vi "toOCU.vi"(8 "error in (no error)":errorcluster, 10 "NotifierReff":T1, 11 "NetworkStreamWriter in":refnum<class "NetworkStreamWriter.lvclass">) -> (0 "error out":errorcluster, 3 "NetworkStreamWriter out":refnum<class "NetworkStreamWriter.lvclass">)   [LabVIEW 2013]
doc: "writes all notifiers to OCU when they're updated\n\nImportaint: when new notifiers are created, this VI must be updated. For doubles, booleans, and double arrays, simply add them to the appropriate unbundle category. For anything else, add them to the \"other\" category and copy the code from the others.\n\nKaitlin Gallagher\n3/4/14"
uses:
  RIO-OCU_Comm/NetworkStreams/Writer/NetworkStreamWriter.lvclass
  Data/TypeDefs/Notifiers.ctl
  Data/TypeDefs/UTM Location.ctl
  Data/TypeDefs/Sail Set Suggestions.ctl
  Data/TypeDefs/Rudder Set Suggestions.ctl
  Data/TypeDefs/OverrideInformation.ctl
  Data/TypeDefs/OverrideMode.ctl
  Data/TypeDefs/MotorSetup.ctl
  Data/TypeDefs/DynamixelSetupInfo.ctl
  Data/TypeDefs/AirmarStatus.ctl
  Data/TypeDefs/HardwareOnline.ctl
  <vilib>/Utility/VariantDataType/VariantType.lvlib
panel:
  out "error in (no error) 3":errorcluster
  in  "error in (no error) 2":errorcluster
  out "latest notification":dbl
  out "Numeric":i32
  out "Array":string[](array[string])
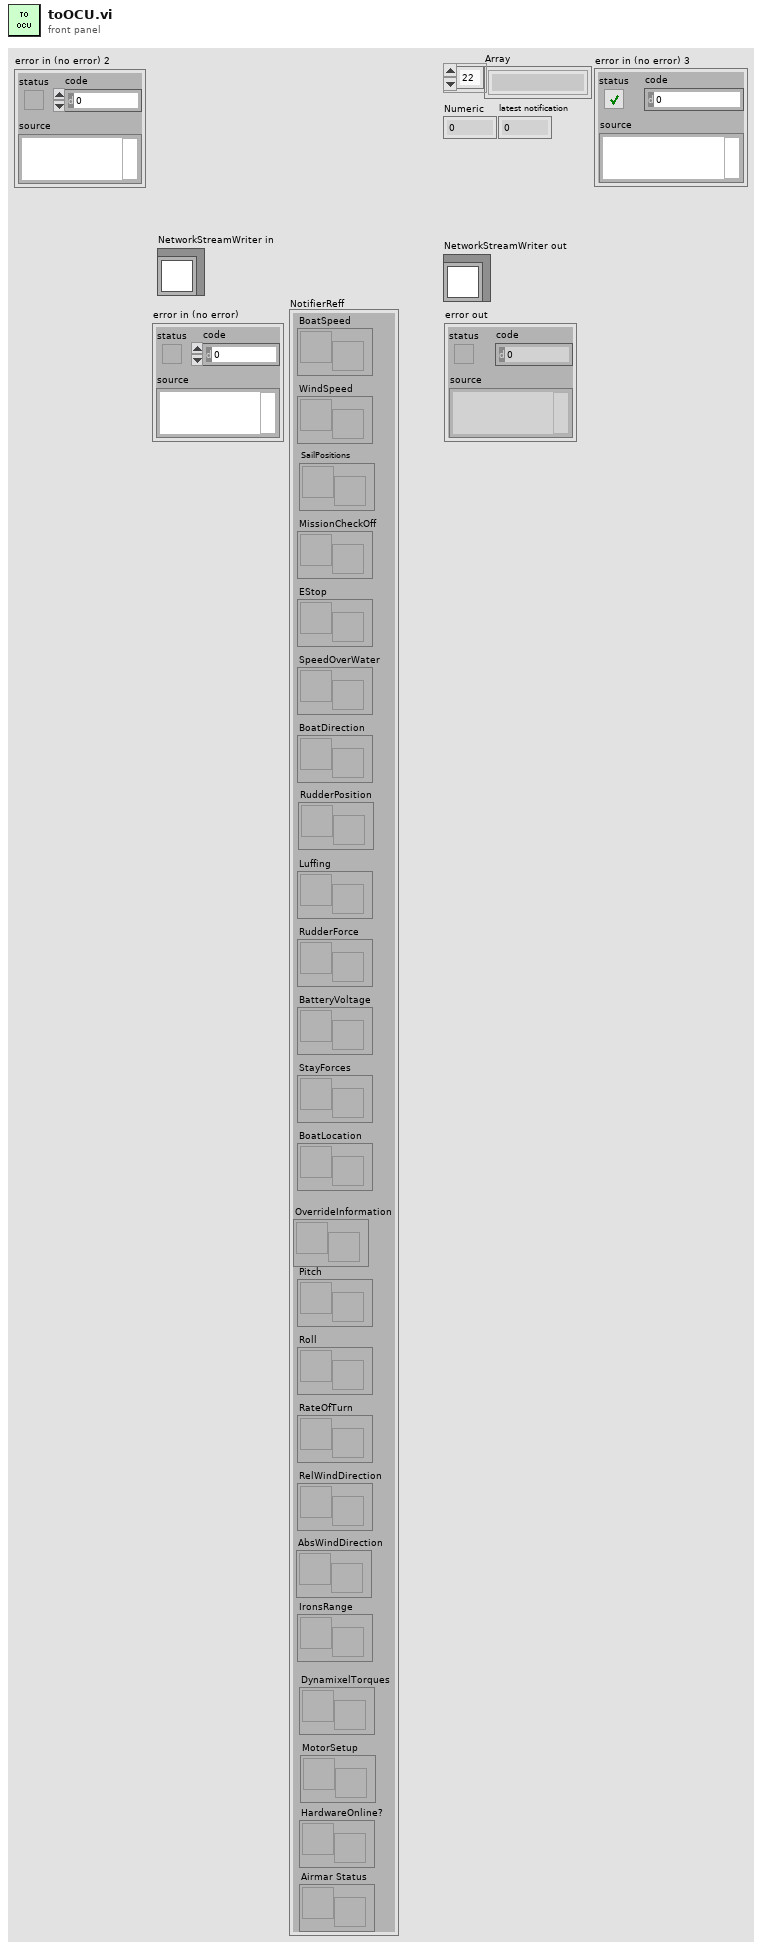
[diagram p1: front panel]
types:
  T1 = typedef "Notifiers.ctl" = cluster{"BoatSpeed":refnum<notifier>, "WindSpeed":refnum<notifier>, "MissionCheckOff":refnum<notifier>, "EStop":refnum<notifier>, "SpeedOverWater":refnum<notifier>, "BoatDirection":refnum<notifier>, "Luffing":refnum<notifier>, "RudderForce":refnum<notifier>, "BatteryVoltage":refnum<notifier>, "StayForces":refnum<notifier>, "BoatLocation":refnum<notifier>, "Pitch":refnum<notifier>, "Roll":refnum<notifier>, "RateOfTurn":refnum<notifier>, "RelWindDirection":refnum<notifier>, "SailPositions":refnum<notifier>, "RudderPosition":refnum<notifier>, "IronsRange":refnum<notifier>, "AbsWindDirection":refnum<notifier>, "OverrideInformation":refnum<notifier>, "DynamixelTorques":refnum<notifier>, "MotorSetup":refnum<notifier>, "Airmar Status":refnum<notifier>, "HardwareOnline?":refnum<notifier>}
  T2 = typedef "HardwareOnline.ctl" = cluster{"AirmarOnline":bool, "WindvaneOnline":bool, "HemisphereOnline":bool, "StayForceOnline":bool, "BatteryVoltageOnline":bool, "AccelerometerOnline":bool, "MainDynamixel Online":bool, "JibDynamixel Online":bool, "RudderDynamixel Online":bool}
  T3 = typedef "MotorSetup.ctl" = cluster{"Main Dynamixel Set Data":T4, "Rudder Dynamixel Set Data":T4, "Jib Dynamixel Set Data":T4}
  T4 = typedef "DynamixelSetupInfo.ctl" = cluster{"Lower Winch Bound":dbl, "Upper Winch Bound":dbl, "Reverse Winch Direction?":bool, "Dynamixel Cycle Number":i32}
  T5 = typedef "OverrideInformation.ctl" = cluster{"OverrideMode":T6, "SailSetting":T7, "Rudder Setpoint":T8}
  T6 = typedef "OverrideMode.ctl" = enum16{"None", "Rudder", "Sails", "Both"}
  T7 = typedef "Sail Set Suggestions.ctl" = cluster{"MainSailSuggestion":dbl, "JibSailSuggestion":dbl}
  T8 = typedef "Rudder Set Suggestions.ctl" = dbl
  T9 = typedef "UTM Location.ctl" = cluster{"UTM Zone":dbl, "Hemisphere":enum16{"North", "South"}, "East":dbl, "North":dbl}
  T10 = typedef "VariantType.lvlib/Type.ctl" = enum8{"Invalid Type", "Void", "I8", "I16", "I32", "I64", "U8", "U16", "U32", "U64", "Single Float", "Double Float", "Extended Float", "Single Complex", "Double Complex", "Extended Complex", "Enum U8", "Enum U16", "Enum U32", "Enum U64", "Single Float With Unit", "Double Float With Unit", "Extended Float With Unit", "Single Complex with Unit", "Double Complex with Unit", "Extended Complex with Unit", "Boolean", "String", "Path", "Picture", "Tag", "Array", "Cluster", "Variant", "LV Variant", "Waveform", "Timestamp", "Digital Waveform", "Digital Data", "ExpressData", "Refnum", "External Data", "VI", "Poly VI", "LabVIEW Class Instance", "Fixed Point"}
  T11 = cluster{"AirmarOnline":bool, "WindvaneOnline":bool, "HemisphereOnline":bool, "RudderForceOnline":bool, "StayForceOnline":bool, "BatteryVoltageOnline":bool, "AccelerometerOnline":bool, "MainDynamixel Online":bool, "JibDynamixel Online":bool, "RudderDynamixel Online":bool}
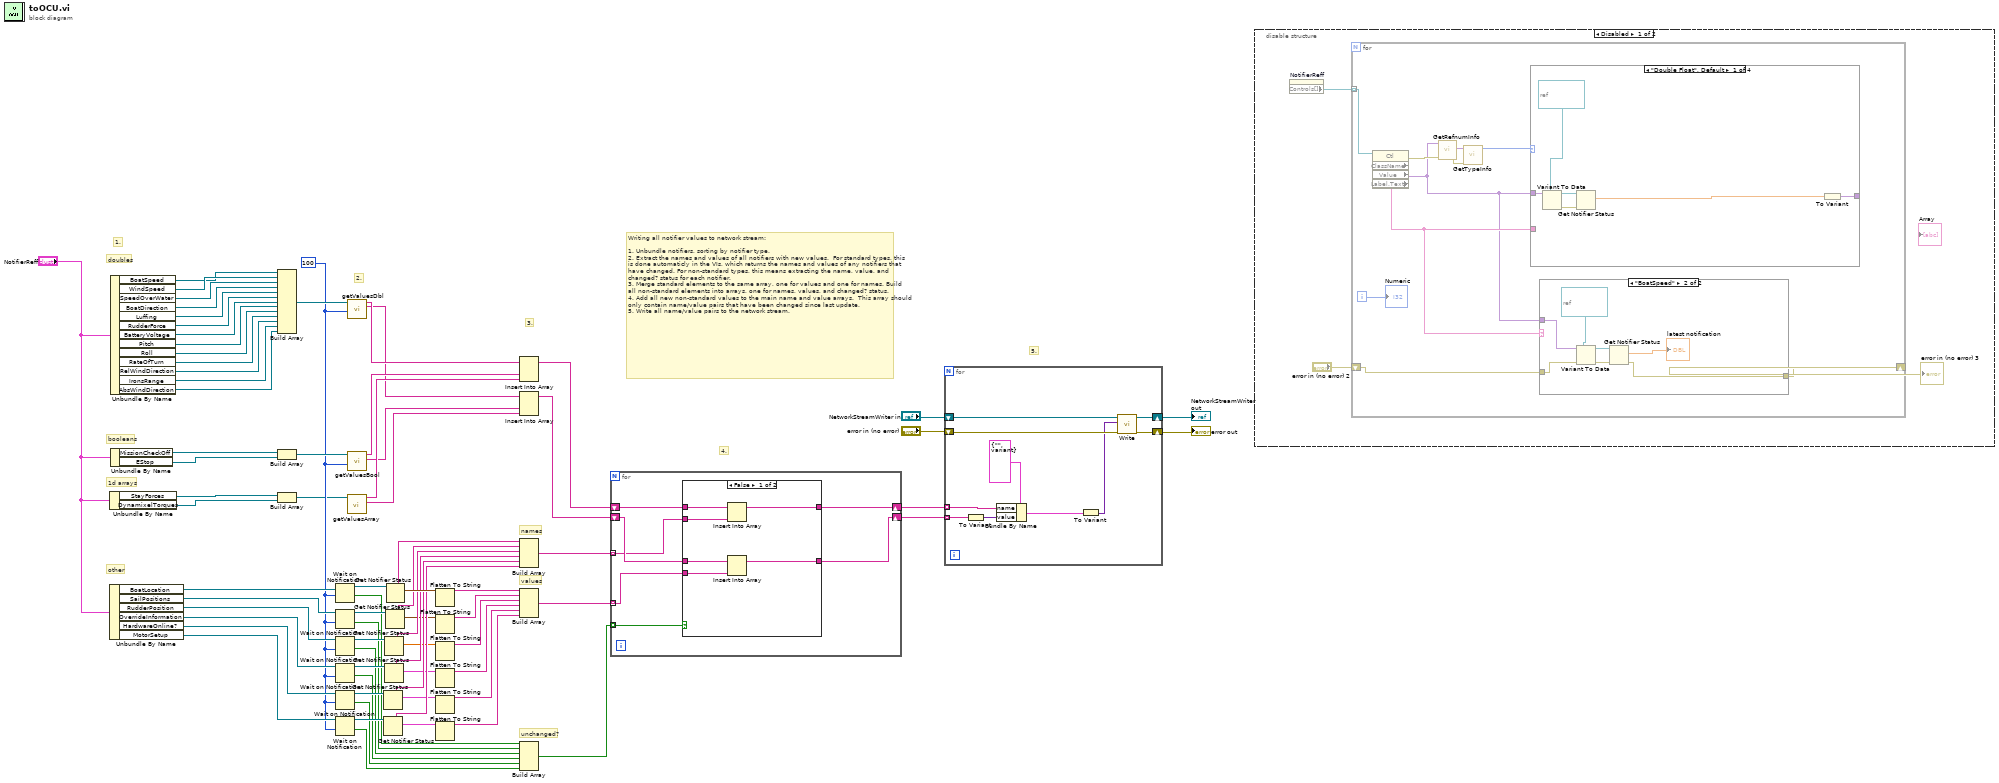
[diagram p0: block diagram]
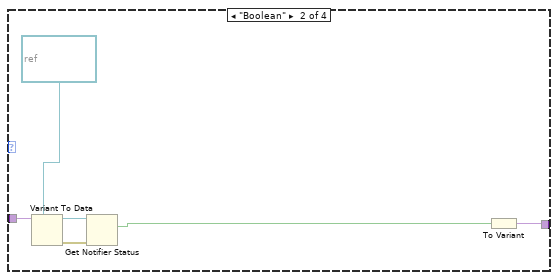
[diagram p3: hidden frame]
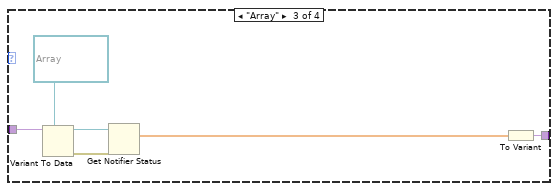
[diagram p4: hidden frame]
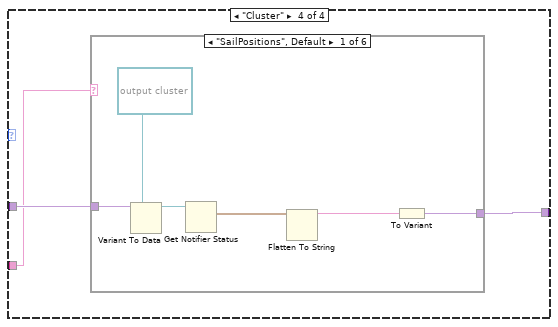
[diagram p5: hidden frame]
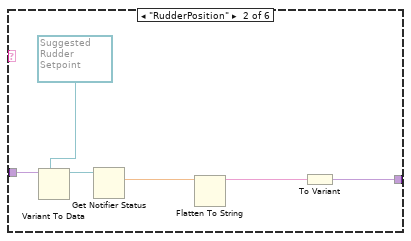
[diagram p6: hidden frame]
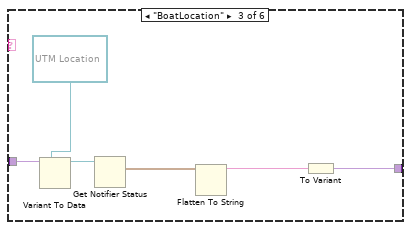
[diagram p7: hidden frame]
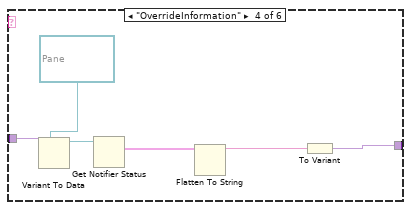
[diagram p8: hidden frame]
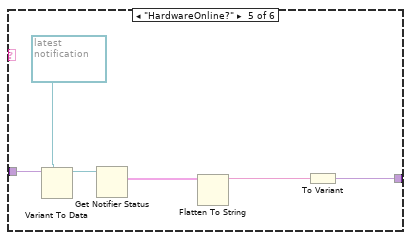
[diagram p9: hidden frame]
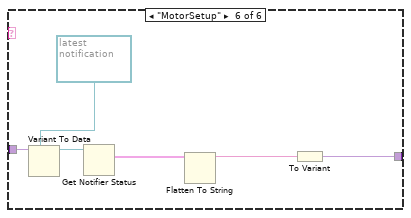
[diagram p10: hidden frame]
diagram:
  w39 = 100 ("timeout in ms (-1)")
  # "Writing all notifier values to network stream:\n\n1. Unbundle notifiers, sorting by notifier type.\n2. Extract the names and values of all notifiers with new values.  For standard types, this is done automaticly in the VIs, which returns the names and values of any notifiers that have changed. For non-standard types, this means extracting the name, value, and changed? status for each notifier. \n3. Merge standard elements to the same array, one for values and one for names. Build all non-standard elements into arrays, one for names, values, and changed? status.\n4. Add all new non-standard values to the main name and value arrays.  This array should only contain name/value pairs that have been changed since last update.\n5. Write all name/value pairs to the network stream."
  # "5."
  # "4."
  # "3."
  # "2."
  # "1."
  # "unchanged?"
  # "values"
  # "names"
  # "other"
  # "1d arrays"
  # "booleans"
  # "doubles"
  n1 = Unbundle By Name("NotifierReff") -> ("StayForces"=w59:refnum<notifier>, "DynamixelTorques"=w62:refnum<notifier>)
  n2 = Unbundle By Name("NotifierReff") -> ("BoatLocation"=w58:refnum<notifier>, "SailPositions"=w57:refnum<notifier>, "RudderPosition"=w56:refnum<notifier>, "OverrideInformation"=w54:refnum<notifier>, "HardwareOnline?"=w55:refnum<notifier>, "MotorSetup"=w53:refnum<notifier>)
  n3 = Unbundle By Name("NotifierReff") -> ("BoatSpeed"=w42:refnum<notifier>, "WindSpeed"=w75:refnum<notifier>, "SpeedOverWater"=w74:refnum<notifier>, "BoatDirection"=w73:refnum<notifier>, "Luffing"=w72:refnum<notifier>, "RudderForce"=w71:refnum<notifier>, "BatteryVoltage"=w70:refnum<notifier>, "Pitch"=w69:refnum<notifier>, "Roll"=w68:refnum<notifier>, "RateOfTurn"=w67:refnum<notifier>, "RelWindDirection"=w66:refnum<notifier>, "IronsRange"=w65:refnum<notifier>, "AbsWindDirection"=w64:refnum<notifier>)
  n4 = Unbundle By Name("NotifierReff") -> ("MissionCheckOff"=w60:refnum<notifier>, "EStop"=w63:refnum<notifier>)
  n5 = Build Array(w42, w75, w74, w73, w72, w71, w70, w69, w68, w67, w66, w65, w64) -> (w41:refnum<notifier>[])
  n6 = Build Array(w60, w63) -> (w40:refnum<notifier>[])
  n7 = Build Array(w59, w62) -> (w38:refnum<notifier>[])
  n8 = Wait on Notification(notifier=w58, timeout in ms (-1)=w39) -> (notifier out=w37:refnum<notifier>, timed out?=w14:bool)  [unwired: 2 in, 2 out]
  n9 = Wait on Notification(notifier=w57, timeout in ms (-1)=w39) -> (notifier out=w34:refnum<notifier>, timed out?=w15:bool)  [unwired: 2 in, 2 out]
  n10 = Wait on Notification(notifier=w56, timeout in ms (-1)=w39) -> (notifier out=w32:refnum<notifier>, timed out?=w16:bool)  [unwired: 2 in, 2 out]
  n11 = Wait on Notification(notifier=w54, timeout in ms (-1)=w39) -> (notifier out=w30:refnum<notifier>, timed out?=w17:bool)  [unwired: 2 in, 2 out]
  n12 = Wait on Notification(notifier=w55, timeout in ms (-1)=w39) -> (notifier out=w28:refnum<notifier>, timed out?=w18:bool)  [unwired: 2 in, 2 out]
  n13 = Wait on Notification(notifier=w53, timeout in ms (-1)=w39) -> (notifier out=w26:refnum<notifier>, timed out?=w19:bool)  [unwired: 2 in, 2 out]
  n14 = call "getValuesArray.vi"("appended array"=w38) -> ("notifier values"=w8:string[], "notifier names"=w11:string[])  [unwired: 8 in, 1 out]
  n15 = call "getValuesDbl.vi"("timeout in ms (-1)"=w39, "notifiers in"=w41) -> ("notifier values"=w10:string[], "notifier names"=w13:string[])  [unwired: 7 in, 1 out]
  n16 = call "getValuesBool.vi"("timeout in ms (-1)"=w39, "notifiers in"=w40) -> ("notifier values"=w9:string[], "notifier names"=w12:string[])  [unwired: 7 in, 1 out]
  n17 = Get Notifier Status(notifier=w28) -> (notifier name=w27:string, current notification=w21:T2)  [unwired: 1 in, 3 out]
  n18 = Get Notifier Status(notifier=w26) -> (notifier name=w25:string, current notification=w20:T3)  [unwired: 1 in, 3 out]
  n19 = Get Notifier Status(notifier=w30) -> (notifier name=w29:string, current notification=w22:T5)  [unwired: 1 in, 3 out]
  n20 = Get Notifier Status(notifier=w32) -> (notifier name=w31:string, current notification=w23:T8)  [unwired: 1 in, 3 out]
  n21 = Get Notifier Status(notifier=w34) -> (notifier name=w33:string, current notification=w24:T7)  [unwired: 1 in, 3 out]
  n22 = Get Notifier Status(notifier=w37) -> (notifier name=w35:string, current notification=w36:T9)  [unwired: 1 in, 3 out]
  n23 = Flatten To String(anything=w36) -> (data string=w52:string)  [unwired: 3 in, 2 out]
  n24 = Flatten To String(anything=w24) -> (data string=w51:string)  [unwired: 3 in, 2 out]
  n25 = Flatten To String(anything=w23) -> (data string=w50:string)  [unwired: 3 in, 2 out]
  n26 = Flatten To String(anything=w22) -> (data string=w49:string)  [unwired: 3 in, 2 out]
  n27 = Flatten To String(anything=w21) -> (data string=w48:string)  [unwired: 3 in, 2 out]
  n28 = Flatten To String(anything=w20) -> (data string=w47:string)  [unwired: 3 in, 2 out]
  n29 = Insert Into Array(array=w13, new element #1=w12, new element #2=w11) -> (w7:string[])  [unwired: 1 in]
  n30 = Insert Into Array(array=w10, new element #1=w9, new element #2=w8) -> (w6:string[])  [unwired: 1 in]
  n31 = Build Array(w35, w33, w31, w29, w27, w25) -> (w4:string[])
  n32 = Build Array(w52, w51, w50, w49, w48, w47) -> (w3:string[])
  n33 = Build Array(w14, w15, w16, w17, w18, w19) -> (w5:bool[])
  n34 = for {
    tunnel: w5 -> [w82] mode=indexing
    shift-right: [w81] -> w2
    shift-left: w7 -> [w76]
    shift-right: [w79] -> w1
    shift-left: w6 -> [w80]
    tunnel: w4 -> [w78] mode=indexing
    tunnel: w3 -> [w77] mode=indexing
    n35 = case shown="False" w82 {
      tunnel: [w88 w89] -> w81
      tunnel: w80 -> [w87 w90]
      tunnel: [w86 w90] -> w79
      tunnel: w78 -> [w85 _]
      tunnel: w77 -> [w84 _]
      tunnel: w76 -> [w83 w89]
      frame False {
        n36 = Insert Into Array(array=w83, new element=w85) -> (w88:string[])  [unwired: 1 in]
        n37 = Insert Into Array(array=w87, new element=w84) -> (w86:string[])  [unwired: 1 in]
      }
      frame True {
      }
    }
  }
  n38 = for {
    shift-right: [w97] -> w43
    shift-left: "error in (no error)" -> [w100]
    shift-right: [w98] -> w44
    shift-left: "NetworkStreamWriter in" -> [w99]
    tunnel: w2 -> [w94] mode=indexing
    tunnel: w1 -> [w92] mode=indexing
    n39 = To Variant(anything=w92) -> (Variant=w91:variant)
    n40 = Bundle By Name(cluster=cluster{"name":string, "value":variant} {"name"="", "value"=variant} ("input cluster"), "name"=w94, "value"=w91) -> (w93:cluster{"name":string, "value":variant})
    n41 = To Variant(anything=w93) -> (Variant=w96:variant)
    n42 = call "Write.vi"("error in (no error)"=w100, "element"=w96, "NetworkStreamWriter in"=w99) -> ("error out"=w97:errorcluster, "NetworkStreamWriter out"=w98:refnum<class "NetworkStreamWriter.lvclass">)  [unwired: 7 in]
  }
  "NetworkStreamWriter out" <- w44
  "error out" <- w43
  n43 = disable-structure shown="Disabled" {
    frame Disabled {
      n44 = property on="NotifierReff" class="Clust (strict)"() -> ("Controls[]"=w103:refnum<vi>[])  [unwired: 2 in, 2 out]
      n45 = for {
        tunnel: w103 -> [w113] mode=indexing
        shift-right: [w104] -> w101
        shift-left: "error in (no error) 2" -> [w105]
        i -> [w108]
        n46 = property class="Ctl" props=["ClassName", "Value", "Label", "Text"](reference=w113) -> (error out=w112:errorcluster, "Value"=w106:variant, "Label.Text"=w107:string)  [unwired: 1 in, 2 out]
        n47 = call <vilib>:"GetRefnumInfo.vi"("error in (no error)"=w112, "Variant"=w106) -> ("error out"=w109:errorcluster, "StrictType"=w111:variant)  [unwired: 6 in, 2 out]
        n48 = call <vilib>:"GetTypeInfo.vi"("error in (no error)"=w109, "Variant"=w111) -> ("Type Enum"=w110:T10)  [unwired: 5 in, 4 out]
        n49 = case shown="\"Double Float\", Default" w110 {
          tunnel: w106 -> [w119 w125 w131 w134]
          tunnel: [w116 w121 w127 w133] -> _
          tunnel: w107 -> [_ _ _ w132]
          frame "Double Float", Default {
            n50 = Variant To Data(type=refnum<notifier> refnum ("BoatSpeed"), Variant=w119) -> (data=w117:refnum<notifier>, error out=w114:errorcluster)  [unwired: 1 in]
            n51 = Get Notifier Status(notifier=w117, error in (no error)=w114) -> (current notification=w115:dbl)  [unwired: 4 out]
            n52 = To Variant(anything=w115) -> (Variant=w116:variant)
          }
          frame "Boolean" {
            n53 = Variant To Data(type=refnum<notifier> refnum ("EStop"), Variant=w125) -> (data=w123:refnum<notifier>, error out=w120:errorcluster)  [unwired: 1 in]
            n54 = Get Notifier Status(notifier=w123, error in (no error)=w120) -> (current notification=w122:bool)  [unwired: 4 out]
            n55 = To Variant(anything=w122) -> (Variant=w121:variant)
          }
          frame "Array" {
            n56 = Variant To Data(type=refnum<notifier> refnum ("StayForces"), Variant=w131) -> (data=w129:refnum<notifier>, error out=w126:errorcluster)  [unwired: 1 in]
            n57 = Get Notifier Status(notifier=w129, error in (no error)=w126) -> (current notification=w128:dbl[])  [unwired: 4 out]
            n58 = To Variant(anything=w128) -> (Variant=w127:variant)
          }
          frame "Cluster" {
            n59 = case shown="\"SailPositions\", Default" w132 {
              tunnel: w134 -> [w140 w144 w150 w156 w162 w168]
              tunnel: [w137 w142 w149 w154 w161 w166] -> w133
              frame "SailPositions", Default {
                n60 = Variant To Data(type=refnum<notifier> refnum ("SailPositions"), Variant=w140) -> (data=w138:refnum<notifier>)  [unwired: 1 in, 1 out]
                n61 = Get Notifier Status(notifier=w138) -> (current notification=w136:T7)  [unwired: 1 in, 4 out]
                n62 = Flatten To String(anything=w136) -> (data string=w135:string)  [unwired: 3 in, 2 out]
                n63 = To Variant(anything=w135) -> (Variant=w137:variant)
              }
              frame "RudderPosition" {
                n64 = Variant To Data(type=refnum<notifier> refnum ("RudderPosition"), Variant=w144) -> (data=w146:refnum<notifier>)  [unwired: 1 in, 1 out]
                n65 = Get Notifier Status(notifier=w146) -> (current notification=w145:T8)  [unwired: 1 in, 4 out]
                n66 = Flatten To String(anything=w145) -> (data string=w141:string)  [unwired: 3 in, 2 out]
                n67 = To Variant(anything=w141) -> (Variant=w142:variant)
              }
              frame "BoatLocation" {
                n68 = Variant To Data(type=refnum<notifier> refnum ("BoatLocation"), Variant=w150) -> (data=w152:refnum<notifier>)  [unwired: 1 in, 1 out]
                n69 = Get Notifier Status(notifier=w152) -> (current notification=w151:T9)  [unwired: 1 in, 4 out]
                n70 = Flatten To String(anything=w151) -> (data string=w147:string)  [unwired: 3 in, 2 out]
                n71 = To Variant(anything=w147) -> (Variant=w149:variant)
              }
              frame "OverrideInformation" {
                n72 = Variant To Data(type=refnum<notifier> refnum ("OverrideInformation"), Variant=w156) -> (data=w158:refnum<notifier>)  [unwired: 1 in, 1 out]
                n73 = Get Notifier Status(notifier=w158) -> (current notification=w157:T5)  [unwired: 1 in, 4 out]
                n74 = Flatten To String(anything=w157) -> (data string=w153:string)  [unwired: 3 in, 2 out]
                n75 = To Variant(anything=w153) -> (Variant=w154:variant)
              }
              frame "HardwareOnline?" {
                n76 = Variant To Data(type=refnum<notifier> refnum ("HardwareOnline?"), Variant=w162) -> (data=w164:refnum<notifier>)  [unwired: 1 in, 1 out]
                n77 = Get Notifier Status(notifier=w164) -> (current notification=w163:T11)  [unwired: 1 in, 4 out]
                n78 = Flatten To String(anything=w163) -> (data string=w159:string)  [unwired: 3 in, 2 out]
                n79 = To Variant(anything=w159) -> (Variant=w161:variant)
              }
              frame "MotorSetup" {
                n80 = Variant To Data(type=refnum<notifier> refnum ("MotorSetup"), Variant=w168) -> (data=w170:refnum<notifier>)  [unwired: 1 in, 1 out]
                n81 = Get Notifier Status(notifier=w170) -> (current notification=w169:T3)  [unwired: 1 in, 4 out]
                n82 = Flatten To String(anything=w169) -> (data string=w165:string)  [unwired: 3 in, 2 out]
                n83 = To Variant(anything=w165) -> (Variant=w166:variant)
              }
            }
          }
        }
        n84 = case shown="\"BoatSpeed\"" w107 {
          tunnel: w106 -> [_ w178]
          tunnel: w105 -> [w171 w174]
          tunnel: [w171 w172] -> w104
          frame "False", Default {
          }
          frame "BoatSpeed" {
            n85 = Variant To Data(error in=w174, type=refnum<notifier> refnum ("BoatSpeed"), Variant=w178) -> (data=w176:refnum<notifier>, error out=w173:errorcluster)
            n86 = Get Notifier Status(notifier=w176, error in (no error)=w173) -> (current notification=→"latest notification":dbl, error out=w172:errorcluster)  [unwired: 3 out]
          }
        }
        "Numeric" <- w108
      }
      "error in (no error) 3" <- w101
    }
    frame Enabled {
    }
  }
